vi "Stop Core.vi"(10 "final error code":i32, 11 "CS++DSCMonitor in":refnum<class "CS++DSCMonitor.lvclass">) -> (3 "CS++DSCMonitor out":refnum<class "CS++DSCMonitor.lvclass">)   [LabVIEW 2014, in "CS++DSCMonitor.lvlib" / "CS++DSCMonitor.lvclass"]
doc: "(<B>Filename</B>: Actor Framework.lvlib:Actor.lvclass:Stop Core.vi)\n\nDefines what the actor does before it stops. Use the <B>final error code</B> input to determine whether the actor shut down in response to an error.\n\nBy default, this method does nothing. A descendant class may override it to define behavior, such as shutting down any processes the actor initiated in its override of the Actor Core method."
uses:
  CS++DSCMonitor.lvclass
  CSPP_Core/Actors/CS++SVMonitor/CS++SVMonitor.lvclass
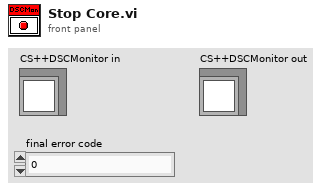
[diagram p1: front panel]
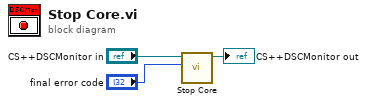
[diagram p0: block diagram]
diagram:
  n1 = call-parent "Stop Core.vi"("final error code"="final error code", "CS++SVMonitor in"="CS++DSCMonitor in") -> ("CS++SVMonitor out"=→"CS++DSCMonitor out":refnum<class "CS++DSCMonitor.lvclass">)  [unwired: 9 in]
